vi "test image custom data.vi"() -> ()   [LabVIEW 2010]
uses:
  <vilib>/vision/driver/IMAQdx.llb/IMAQdx Attribute Type.ctl
  Program Files/National Instruments/LabVIEW 2010/resource/objmgr/imaqdx.rc
  <vilib>/vision/driver/NI_Vision_Acquisition_Software.lvlib
panel:
  out "ValueI64":i64
  out "IncI64":i64
  out "Attribute Information Array":T2(array[cluster])
  out "Description":string
  out "Array":T3(array[cluster])
  out "Keys":string[](array[string])
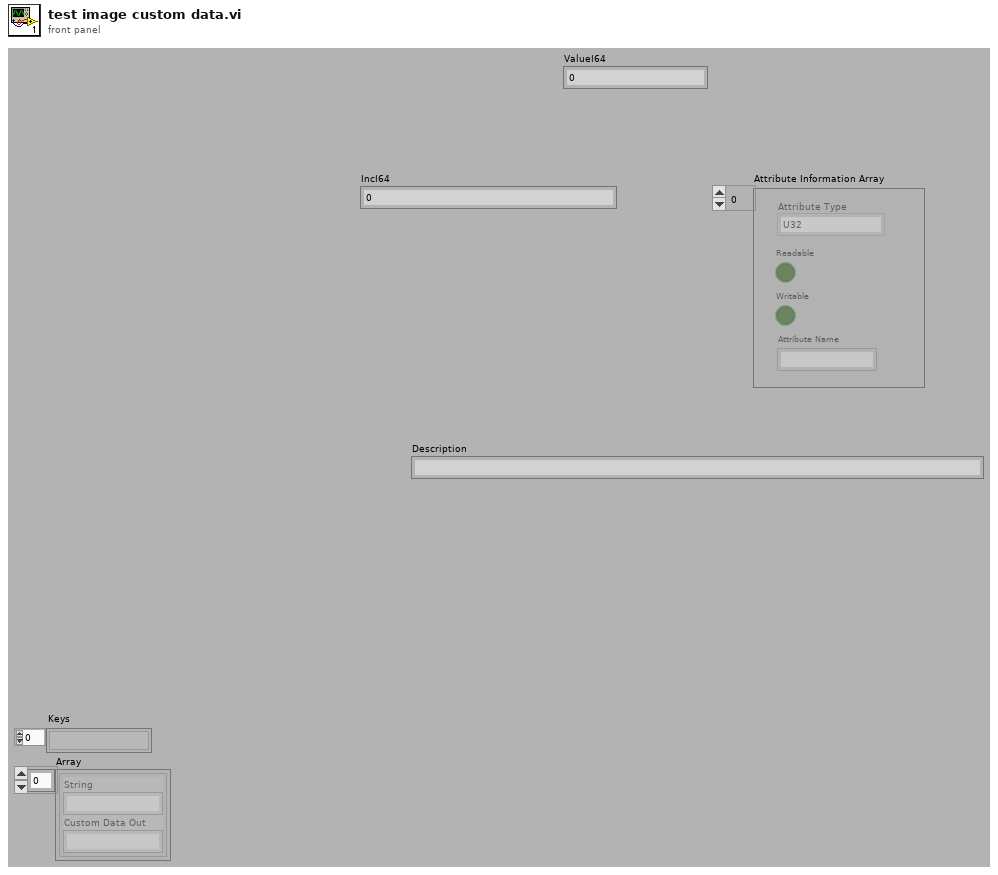
[diagram p1: front panel]
types:
  T1 = typedef "NI_Vision_Acquisition_Software.lvlib/IMAQdx Attribute Type.ctl" = enum32{"U32", "I64", "DBL", "String", "Enum", "Bool", "Command"}
  T2 = cluster{"Attribute Type":T1, "Readable":bool, "Writable":bool, "Attribute Name":string}[]
  T3 = cluster{"String":string, "Custom Data Out":string}[]
  T4 = typedef "IMAQdx.ctl" = refnum<k21>
  T5 = cluster{"Aquisition Type":enum16{"IMAQ", "IMAQdx", "AVI", "MMF", "STACK"}, "Interface Name":string, "use roi":bool, "ROI":cluster{"left":u16, "top":u16, "width":u16, "height":u16}, "camera name":T4, "AVI Path":path, "mmf path":path, "stub":string, "Field Width (0 disables 0 padding)":u8, "extension":string, "inter-frame interval (ms)":dbl}
  T6 = typedef "AviRefnum.ctl" = refnum<k1>
  T7 = typedef "IMAQ Image.ctl" = refnum<image>
  T8 = cluster{"Aquisition Type":enum16{"IMAQ", "IMAQdx", "AVI", "MMF", "STACK"}, "IMAQ Session Out":refnum<k11>, "imaqdx session":T4, "AVI parameters":cluster{"Avi Refnum ":T6, "inter-frame interval (ms)":dbl}, "mmf parameters":cluster{"mmf pointer":u32, "inter-frame interval (ms)":dbl}, "stack read info":cluster{"file stub":string, "format string":string, "extension":string, "inter-frame interval (ms)":dbl}, "camera image":T7, "camera image is 8 bit":bool, "8 bit camera image":T7}
  T9 = cluster{"String":string, "Custom Data Out":string}
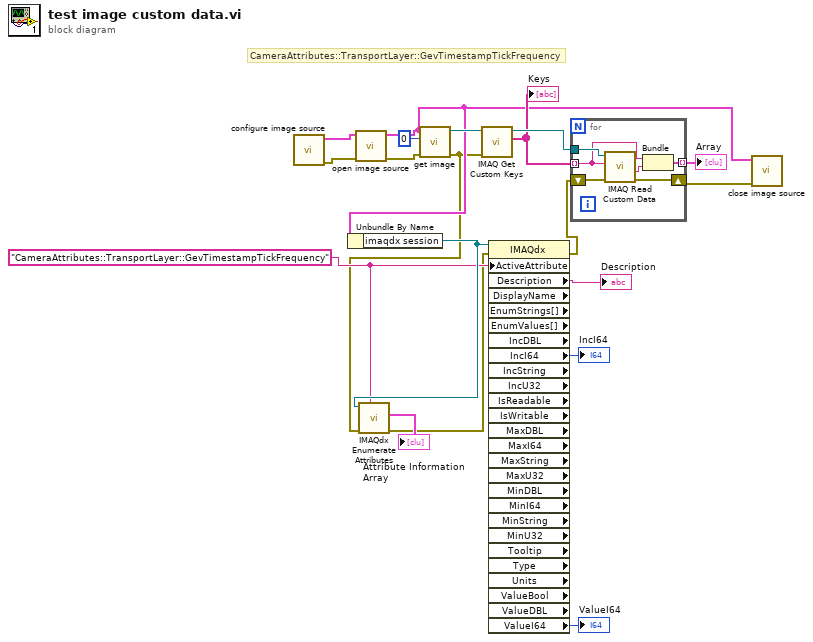
[diagram p0: block diagram]
diagram:
  w6 = "CameraAttributes::TransportLayer::GevTimestampTickFrequency"
  # "CameraAttributes::TransportLayer::GevTimestampTickFrequency"
  n1 = call "configure image source.vi"() -> ("error out"=w19:errorcluster, "image source parameters"=w18:T5)  [unwired: 10 in]
  n2 = call "open image source.vi"("error in (no error)"=w19, "image source parameters"=w18) -> ("error out"=w17:errorcluster, "image source data"=w10:T8)  [unwired: 8 in]
  n3 = Unbundle By Name(w10) -> ("imaqdx session"=w7:T4)
  n4 = call "get image.vi"("error in (no error)"=w17, "previous buffer number"=u32 0, "image source data"=w10) -> ("error out"=w5:errorcluster, "captured image"=w15:T7)  [unwired: 5 in, 2 out]
  n5 = call <vilib>:"IMAQdx Enumerate Attributes.vi"("Root"=w6, "error in"=w5, "Session In"=w7) -> ("error out"=w3:errorcluster, "Attribute Information Array"=→"Attribute Information Array":T2)  [unwired: 6 in, 1 out]
  n6 = call "IMAQ Get Custom Keys"("error in (no error)"=w5, "Image"=w15) -> ("Keys"=w13:string[], "Image (duplicate)"=w14:T7)  [unwired: 6 in, 2 out]
  "Keys" <- w13
  n7 = property class="IMAQdx" props=["ActiveAttribute", "Description", "DisplayName", "EnumStrings[]", "EnumValues[]", "IncDBL", "IncI64", "IncString", "IncU32", "IsReadable", "IsWritable", "MaxDBL", "MaxI64", "MaxString", "MaxU32", "MinDBL", "MinI64", "MinString", "MinU32", "Tooltip", "Type", "Units", "ValueBool", "ValueDBL", "ValueI64"](reference=w7, error in=w3, "ActiveAttribute"=w6) -> (error out=w8:errorcluster, "Description"=→"Description":string, "IncI64"=→"IncI64":i64, "ValueI64"=→"ValueI64":i64)  [unwired: 22 out]
  n8 = for {
    shift-right: [w20] -> w11
    shift-left: w8 -> [w25]
    tunnel: w14 -> [w24]
    tunnel: w13 -> [w22] mode=indexing
    tunnel: [w21] -> w12 mode=indexing
    n9 = call "IMAQ Read Custom Data"("error in (no error)"=w25, "Key"=w22, "Image"=w24) -> ("error out"=w20:errorcluster, "Custom Data Out"=w23:string)  [unwired: 6 in, 1 out]
    n10 = Bundle("String"=w22, "Custom Data Out"=w23) -> (w21:T9)  [unwired: 1 in]
  }
  "Array" <- w12
  n11 = call "close image source.vi"("error in (no error)"=w11, "image source data"=w10) -> ()  [unwired: 9 in, 1 out]
